vi "Trying To Read.vi"() -> ()   [LabVIEW 2020]
uses:
  <vilib>/DAQmx/read.llb/DAQmx Read (Analog 2D DBL NChan NSamp).vi
  <vilib>/DAQmx/create/channels.llb/DAQmx Create Channel (AI-Temperature-Thermocouple).vi
  <vilib>/DAQmx/configure/timing.llb/DAQmx Timing (Sample Clock).vi
  <vilib>/DAQmx/miscellaneous.llb/DAQmx Fill In Error Info.vi
panel:
  in  "stop 2":bool
  out "Waveform Graph 2":dbl[][](graph)
  out "Waveform Graph":dbl[][](graph)
  in  "stop":bool
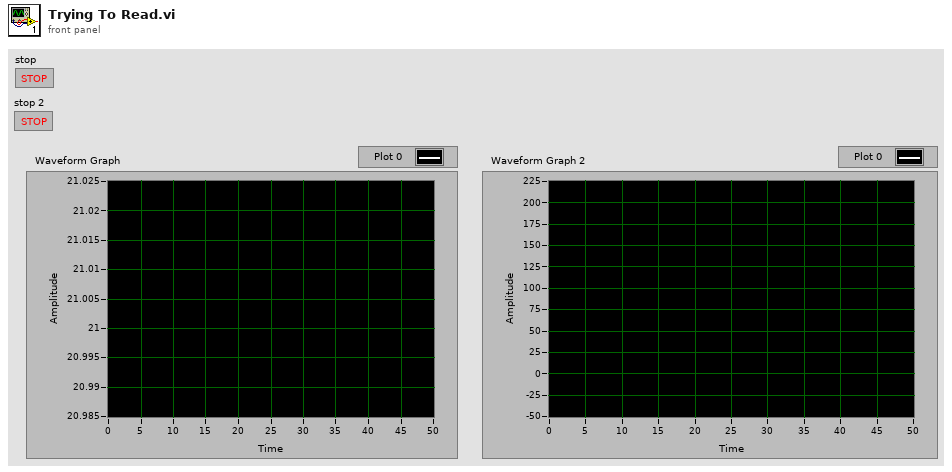
[diagram p1: front panel]
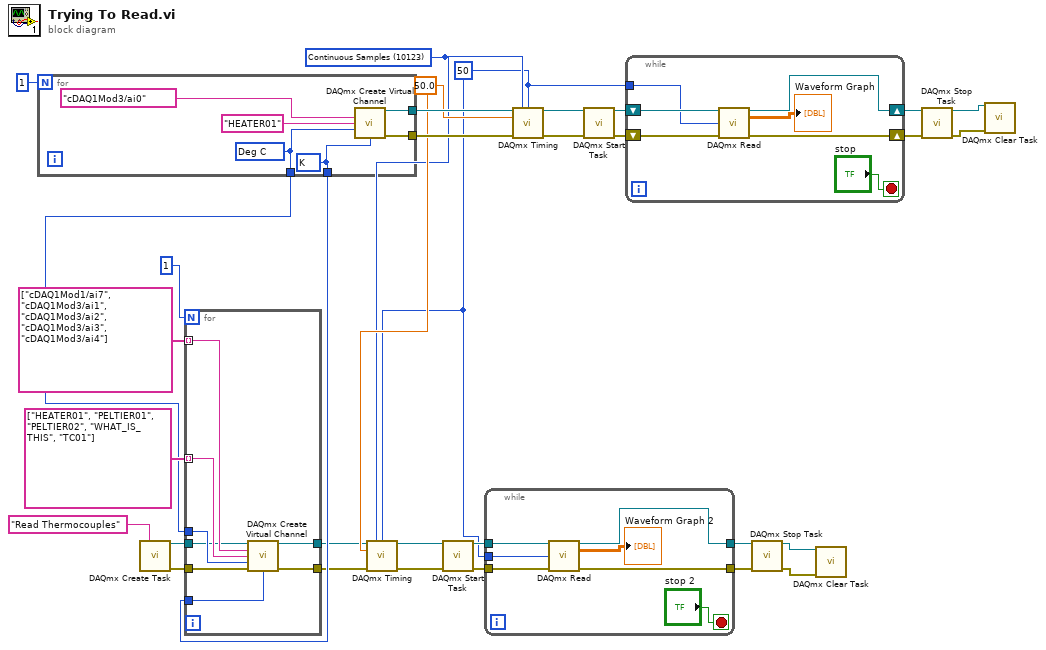
[diagram p0: block diagram]
diagram:
  w7 = 50 ("samples per channel")
  w17 = 10123 items=["Finite Samples"=10178, "Continuous Samples"=10123, "Hardware Timed Single Point"=12522] ("sample mode")
  w22 = 50.0 ("rate")
  n1 = for {
    N: 1 -> [_]
    tunnel: [w38] -> w26
    tunnel: [w37] -> w25
    tunnel: [w34] -> w21
    tunnel: [w33] -> w20
    w34 = 10143 items=["Deg C"=10143, "Deg F"=10144, "Kelvins"=10325, "Deg R"=10145, "From Custom Scale"=10065] ("units")
    w33 = 10073 items=["J"=10072, "K"=10073, "N"=10077, "R"=10082, "S"=10085, "T"=10086, "B"=10047, "E"=10055] ("thermocouple type")
    n2 = call-poly <vilib>:"DAQmx Create Virtual Channel.vi"("physical channels"=tag "cDAQ1Mod3/ai0", "name to assign"="HEATER01", "units"=w34, "thermocouple type"=w33) -> ("task out"=w38:refnum<k21>, "error out"=w37:errorcluster)  [unwired: 10 in]
  }
  n3 = call <vilib>:"DAQmx Create Task.vi"("new task name"="Read Thermocouples") -> ("task out"=w15:refnum<k21>, "error out"=w8:errorcluster)  [unwired: 13 in]
  n4 = for {
    N: 1 -> [_]
    tunnel: tag[] ["cDAQ1Mod1/ai7", "cDAQ1Mod3/ai1", "cDAQ1Mod3/ai2", "cDAQ1Mod3/ai3", "cDAQ1Mod3/ai4"] -> [w46] mode=indexing
    tunnel: string[] ["HEATER01", "PELTIER01", "PELTIER02", "WHAT_IS_THIS", "TC01"] -> [w45] mode=indexing
    tunnel: w21 -> [w44]
    tunnel: w20 -> [w43]
    tunnel: w15 -> [w42]
    tunnel: [w41] -> w12
    tunnel: [w40] -> w9
    tunnel: w8 -> [w39]
    n5 = call-poly <vilib>:"DAQmx Create Virtual Channel.vi"("task in"=w42, "physical channels"=w46, "name to assign"=w45, "units"=w44, "error in"=w39, "thermocouple type"=w43) -> ("task out"=w41:refnum<k21>, "error out"=w40:errorcluster)  [unwired: 8 in]
  }
  n6 = call-poly <vilib>:"DAQmx Timing.vi"("task/channels in"=w12, "sample mode"=w17, "samples per channel"=w7, "rate"=w22, "error in"=w9) -> ("task out"=w11:refnum<k21>, "error out"=w10:errorcluster)  [unwired: 9 in]
  n7 = call <vilib>:"DAQmx Start Task.vi"("task/channels in"=w11, "error in"=w10) -> ("task out"=w14:refnum<k21>, "error out"=w13:errorcluster)  [unwired: 12 in]
  n8 = while {
    tunnel: [w52] -> w19
    tunnel: [w53] -> w18
    tunnel: w14 -> [w49]
    tunnel: w13 -> [w48]
    tunnel: w7 -> [w47]
    stop <- "stop 2" stop-if-true
    n9 = call-poly <vilib>:"DAQmx Read.vi"("task/channels in"=w49, "number of samples per channel"=w47, "error in"=w48) -> ("task out"=w52:refnum<k21>, "data"=→"Waveform Graph 2":dbl[][], "error out"=w53:errorcluster)  [unwired: 10 in]
  }
  n10 = call-poly <vilib>:"DAQmx Timing.vi"("task/channels in"=w26, "sample mode"=w17, "samples per channel"=w7, "rate"=w22, "error in"=w25) -> ("task out"=w28:refnum<k21>, "error out"=w27:errorcluster)  [unwired: 9 in]
  n11 = call <vilib>:"DAQmx Start Task.vi"("task/channels in"=w28, "error in"=w27) -> ("task out"=w32:refnum<k21>, "error out"=w31:errorcluster)  [unwired: 12 in]
  n12 = while {
    shift-right: [w57] -> w29
    shift-left: w32 -> [w60]
    shift-right: [w58] -> w30
    shift-left: w31 -> [w59]
    tunnel: w7 -> [w54]
    stop <- "stop" stop-if-true
    n13 = call-poly <vilib>:"DAQmx Read.vi"("task/channels in"=w60, "number of samples per channel"=w54, "error in"=w59) -> ("task out"=w57:refnum<k21>, "data"=→"Waveform Graph":dbl[][], "error out"=w58:errorcluster)  [unwired: 10 in]
  }
  n14 = call <vilib>:"DAQmx Stop Task.vi"("task/channels in"=w19, "error in"=w18) -> ("task out"=w2:refnum<k21>, "error out"=w1:errorcluster)  [unwired: 12 in]
  n15 = call <vilib>:"DAQmx Clear Task.vi"("task in"=w2, "error in"=w1) -> ()  [unwired: 13 in, 1 out]
  n16 = call <vilib>:"DAQmx Stop Task.vi"("task/channels in"=w29, "error in"=w30) -> ("task out"=w4:refnum<k21>, "error out"=w3:errorcluster)  [unwired: 12 in]
  n17 = call <vilib>:"DAQmx Clear Task.vi"("task in"=w4, "error in"=w3) -> ()  [unwired: 13 in, 1 out]
